vi "Call Set Origin user dialogue.vi"(8 "error in (no error)":errorcluster) -> (0 "error out":errorcluster)   [LabVIEW 2020]
uses:
  Typedefs/XYZ stage states.ctl
  Typedefs/XYZ stage data.ctl
  Typedefs/XYZ channel ring.ctl
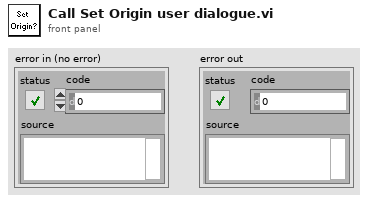
[diagram p1: front panel]
types:
  T1 = typedef "XYZ channel ring.ctl" = string
  T2 = typedef "XYZ stage data.ctl" = cluster{"Command":T3, "Channel":T1, "X":sgl, "Y":sgl, "Z":sgl, "Speed":i32, "Zero":bool, "Use acknowledgement?":bool}
  T3 = typedef "XYZ stage states.ctl" = enum16{"Dequeue", "Initialize", "Read Position", "Read Speed Setting", "Move", "Set Max Speed", "Reset Axis", "Stop all movement"}
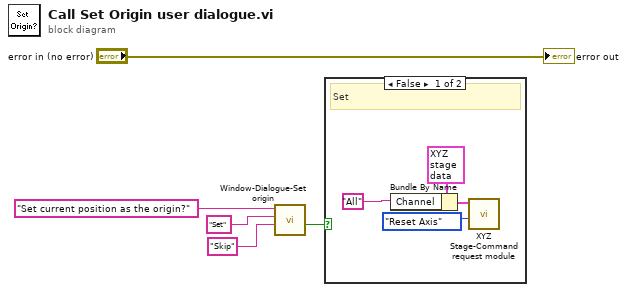
[diagram p0: block diagram]
diagram:
  n1 = call "Window-Dialogue-Set origin.vi"("Caption-Left button (Cancel)"="Skip" ("Caption-Left button"), "Caption-Right button (OK)"="Set" ("Caption-Right button"), "Message string"="Set current position as the origin?") -> ("Cancelled (Left button pressed)"=w1:bool)  [unwired: 7 in, 1 out]
  n2 = case shown="False" w1 {
    frame False {
      # "Set"
      n3 = Bundle By Name(cluster=T2 {"Command"=enum."Initialize", "Channel"="", "X"=0.0, "Y"=0.0, "Z"=0.0, "Speed"=0, "Zero"=FALSE, "Use acknowledgement?"=FALSE} ("XYZ Stage data to queue"), "Channel"=T1 "All") -> (w9:T2)
      n4 = call "XYZ Stage-Command request module.vi"("Command"=XYZ_stage_states."Reset Axis", "XYZ Stage data to queue"=w9) -> ()  [unwired: 5 in, 5 out]
    }
    frame True {
      # "Skip"
    }
  }
  "error out" <- "error in (no error)"
